vi "IsValidHexCode.vi"(1 "Input string":string) -> (0 "Valid":bool)   [LabVIEW 2014]
uses:
  States.ctl
panel:
  out "STATE":T1
  out "RADIX":enum16{"Undefined", "HEX", "BIN", "OCT"}(ring)
  out "unsigned byte array":u8[](array[numeric]) format="%.0x"
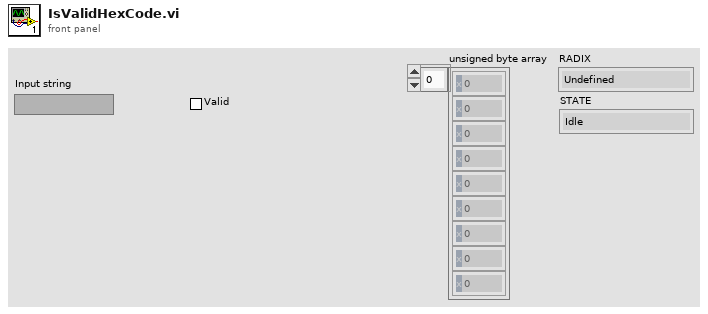
[diagram p1: front panel]
types:
  T1 = typedef "States.ctl" = enum16{"Idle", "Parse radix", "Parse body HEX", "Parse body OCT", "Parse body BIN", "Error"}
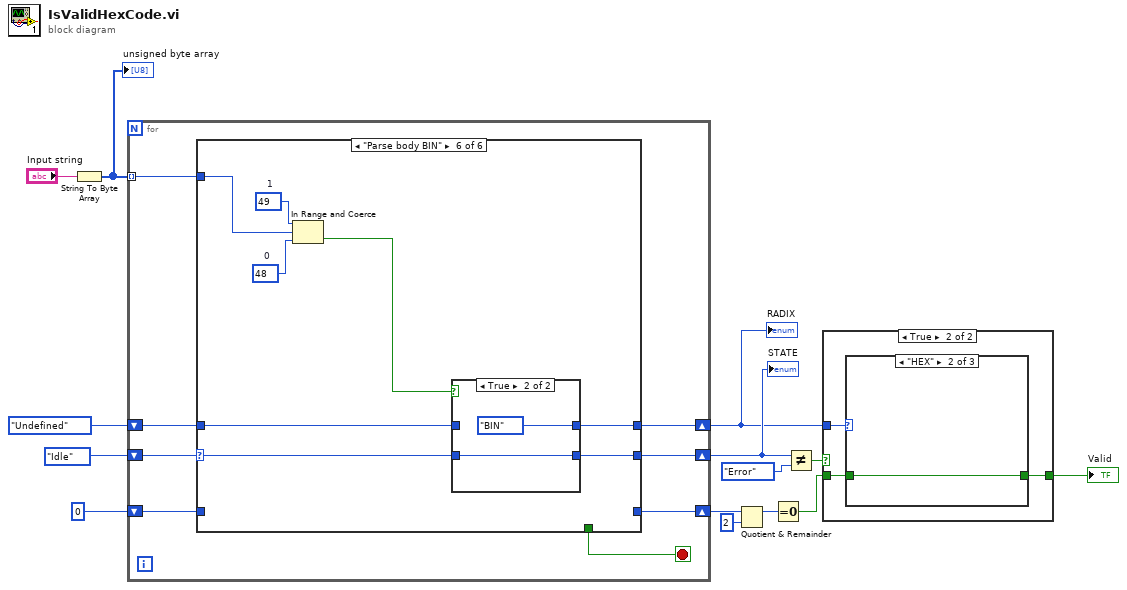
[diagram p0: block diagram]
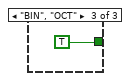
[diagram p4: hidden frame]
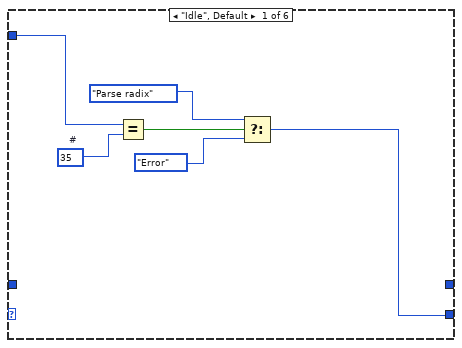
[diagram p5: hidden frame]
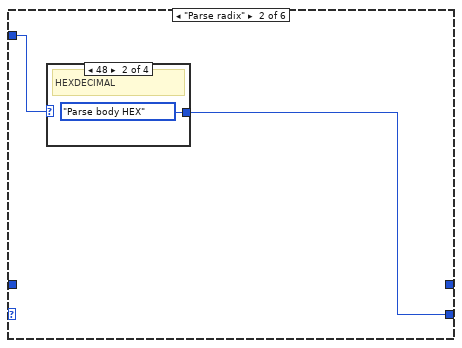
[diagram p6: hidden frame]
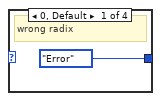
[diagram p7: hidden frame]
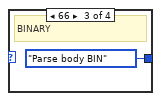
[diagram p8: hidden frame]
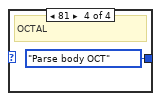
[diagram p9: hidden frame]
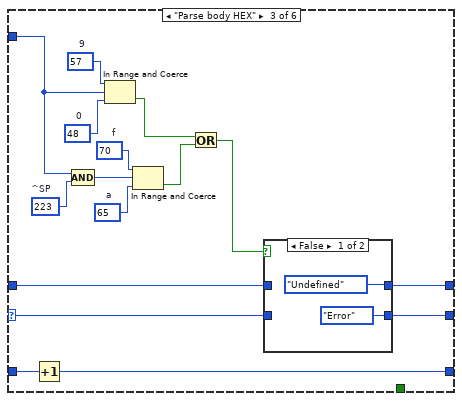
[diagram p10: hidden frame]
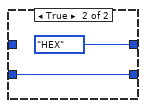
[diagram p11: hidden frame]
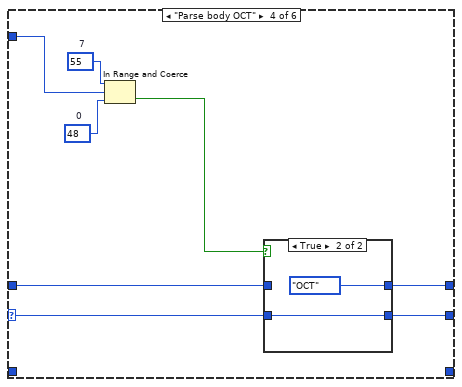
[diagram p12: hidden frame]
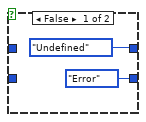
[diagram p13: hidden frame]
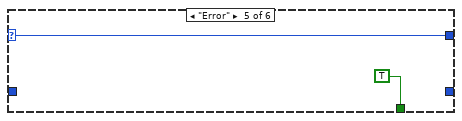
[diagram p14: hidden frame]
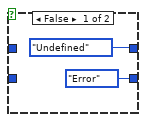
[diagram p15: hidden frame]
diagram:
  n1 = String To Byte Array(string="Input string") -> (unsigned byte array=w13:u8[])
  "unsigned byte array" <- w13
  n2 = for {
    tunnel: w13 -> [w22] mode=indexing
    shift-right: [w20] -> w6
    shift-left: States."Idle" -> [w21]
    shift-right: [w18] -> w3
    shift-left: enum16{"Undefined", "HEX", "BIN", "OCT"}."Undefined" -> [w19]
    shift-right: [w15] -> w9
    shift-left: 0 -> [w16]
    stop <- w17 stop-if-true
    n3 = case shown="\"Parse body BIN\"" w21 {
      selector: w21 -> [_ _ w39 w58 w67 w72]
      tunnel: w22 -> [w27 w30 w48 w60 _ w74]
      tunnel: [w26 w29 w38 w57 w67 w71] -> w20
      tunnel: w19 -> [_ _ w40 w59 _ w73]
      tunnel: [_ _ w37 w56 _ w70] -> w18
      tunnel: [_ _ _ _ TRUE _] -> w17
      tunnel: w16 -> [_ _ w36 _ _ _]
      tunnel: [_ _ w35 _ _ _] -> w15
      frame "Idle", Default {
        w23 = u8 35  # #
        n4 = Equal?(x=w27, y=w23) -> (x = y?=w28:bool)
        n5 = Select(t=States."Parse radix", s=w28, f=States."Error") -> (s? t:f=w26:T1)
      }
      frame "Parse radix" {
        n6 = case shown="48" w30 {
          tunnel: [States."Error" States."Parse body HEX" States."Parse body BIN" States."Parse body OCT"] -> w29
          frame 0, Default {
            # "wrong radix"
          }
          frame 72 {
            # "HEXDECIMAL"
          }
          frame 66 {
            # "BINARY"
          }
          frame 81 {
            # "OCTAL"
          }
        }
      }
      frame "Parse body HEX" {
        w44 = u8 65  # a
        w45 = u8 70  # f
        w47 = u8 223  # ^SP
        w49 = u8 48  # 0
        w50 = u8 57  # 9
        n7 = Increment(x=w36) -> (x+1=w35:i32)
        n8 = Compound Arithmetic op=AND(w48, w47) -> (w46:u8)
        n9 = In Range and Coerce(upper limit=w50, x=w48, lower limit=w49) -> (In Range?=w43:bool)  [unwired: 1 out]
        n10 = In Range and Coerce(upper limit=w45, x=w46, lower limit=w44) -> (In Range?=w42:bool)  [unwired: 1 out]
        n11 = Or(x=w43, y=w42) -> (x .or. y?=w41:bool)
        n12 = case shown="False" w41 {
          tunnel: w40 -> [_ _]
          tunnel: w39 -> [_ w54]
          tunnel: [States."Error" w54] -> w38
          tunnel: [enum16{"Undefined", "HEX", "BIN", "OCT"}."Undefined" enum16{"Undefined", "HEX", "BIN", "OCT"}."HEX"] -> w37
          frame False {
          }
          frame True {
          }
        }
      }
      frame "Parse body OCT" {
        w61 = u8 48  # 0
        w62 = u8 55  # 7
        n13 = In Range and Coerce(upper limit=w62, x=w60, lower limit=w61) -> (In Range?=w55:bool)  [unwired: 1 out]
        n14 = case shown="True" w55 {
          tunnel: w59 -> [_ _]
          tunnel: w58 -> [_ w66]
          tunnel: [States."Error" w66] -> w57
          tunnel: [enum16{"Undefined", "HEX", "BIN", "OCT"}."Undefined" enum16{"Undefined", "HEX", "BIN", "OCT"}."OCT"] -> w56
          frame False {
          }
          frame True {
          }
        }
      }
      frame "Error" {
      }
      frame "Parse body BIN" {
        w75 = u8 48  # 0
        w76 = u8 49  # 1
        n15 = In Range and Coerce(upper limit=w76, x=w74, lower limit=w75) -> (In Range?=w69:bool)  [unwired: 1 out]
        n16 = case shown="True" w69 {
          tunnel: w73 -> [_ _]
          tunnel: w72 -> [_ w80]
          tunnel: [States."Error" w80] -> w71
          tunnel: [enum16{"Undefined", "HEX", "BIN", "OCT"}."Undefined" enum16{"Undefined", "HEX", "BIN", "OCT"}."BIN"] -> w70
          frame False {
          }
          frame True {
          }
        }
      }
    }
  }
  "RADIX" <- w3
  "STATE" <- w6
  n17 = Quotient & Remainder(x=w9, y=2) -> (x-y*floor(x/y)=w7:i32)  [unwired: 1 out]
  n18 = Equal To 0?(x=w7) -> (x = 0?=w2:bool)
  n19 = Not Equal?(x=w6, y=States."Error") -> (x != y?=w4:bool)
  n20 = case shown="True" w4 {
    tunnel: w3 -> [_ w83]
    tunnel: w2 -> [_ w82]
    tunnel: [_ w81] -> w1
    frame False {
    }
    frame True {
      n21 = case shown="\"HEX\"" w83 {
        tunnel: w82 -> [_ w84 _]
        tunnel: [_ w84 TRUE] -> w81
        frame "Undefined", Default {
        }
        frame "HEX" {
        }
        frame "BIN", "OCT" {
        }
      }
    }
  }
  "Valid" <- w1
